vi "ExNCLMult.vi"() -> ()   [LabVIEW 2010]
panel:
  out "Voltage 3":dbl format="%.2f"
  out "Voltage 2":dbl format="%.2f"
  in  "stop":bool
  in  "Number of Detectors (only available for NCL)":u32=1 min=1 max=3 step=1
  in  "Num of Reads to average":u32=1 min=1 step=1
  in  "Gain Range":u32 max=4 step=1
  in  "Integraion / Exposure ms":dbl=1.0 min=1.0 step=1.0 format="%.2f"
  in  "Detector Type":u32=1 min=1 max=3 step=1
  in  "Bi Polar Enable":bool
  in  "High Volts":dbl format="%.2f"
  in  "High Volts Enable":bool
  out "Detector Type":u32
  out "Bi Polar":bool
  out "Gain Value":dbl format="%.2f"
  out "Gain Range":dbl format="%.2f"
  out "Integraion time ms":dbl format="%.2f"
  out "HV Status":bool
  out "HV Volts":dbl format="%.2f"
  out "Get Ave Rds":u32
  out "reserve 2":u32
  out "reserve 1":u32
  out "Voltage 1":dbl format="%.2f"
  out "error out":errorcluster
  in  "error in (no error)":errorcluster
  # "ExNCLMult.vi : shows how to\ncontrol 3 voltages at one time"
  # "1 :  Current\n 2 :  Voltage\n 3 :  Photon Counting"
  # "Minimum is 1.0 ms\nPractical minimum 10.0 ms\nTypical 100.0 ms\nmaximum is 65 sec (65535ms)"
  # "0 : 1x\n1 :  2x\n2 :  4x\n3 : 50x\n4 : 200x"
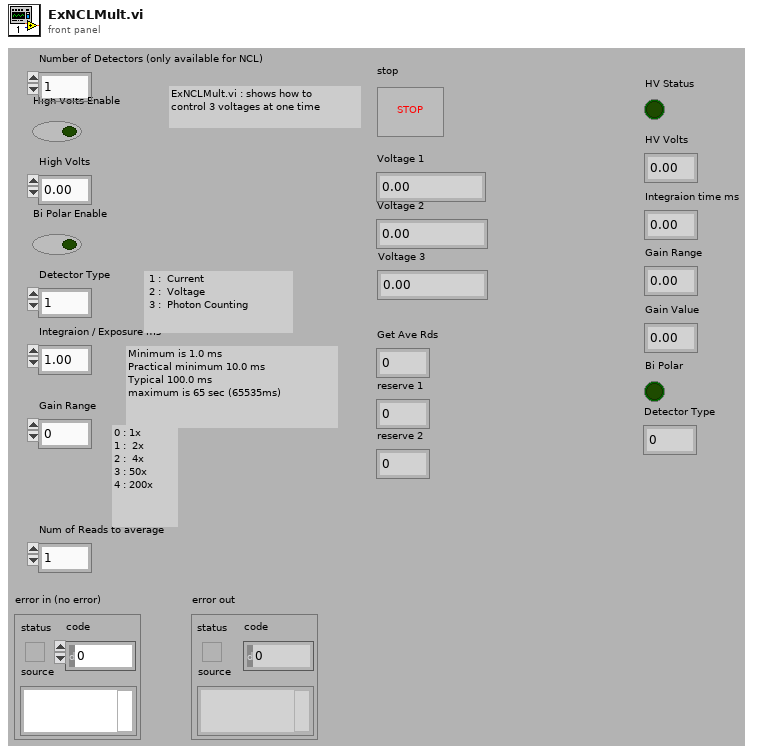
[diagram p1: front panel]
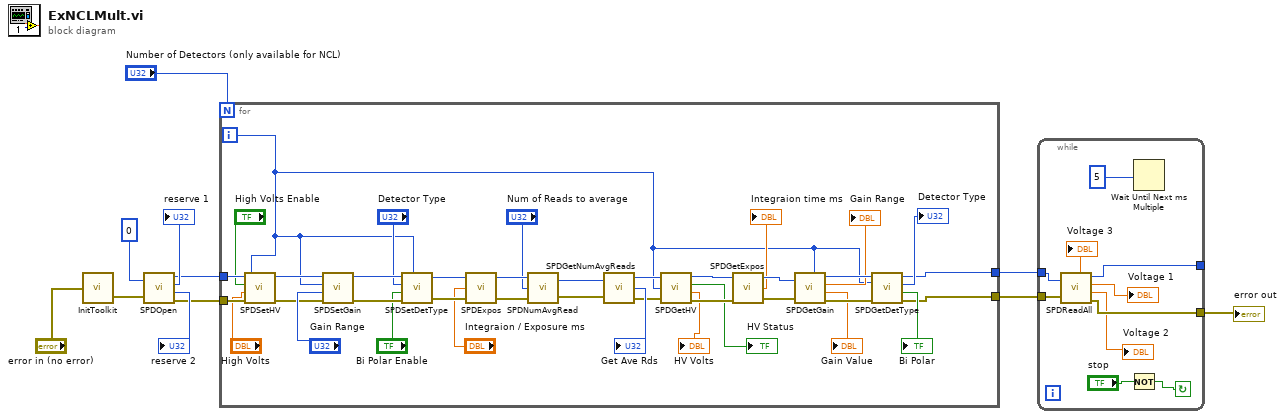
[diagram p0: block diagram]
diagram:
  n1 = call <userlib>:"InitToolkit.vi"("error in"="error in (no error)") -> ("error out"=w10:errorcluster)
  n2 = call <userlib>:"SPDOpen.vi"("Device ID"=0, "error in (no error)"=w10) -> ("SPD Handle"=w5:u32, "reserved 1"=→"reserve 1":u32, "reserved 2"=→"reserve 2":u32, "error out"=w6:errorcluster)
  n3 = for {
    N: "Number of Detectors (only available for NCL)" -> [_]
    tunnel: w6 -> [w33]
    tunnel: w5 -> [w32]
    tunnel: [w14] -> w4
    tunnel: [w13] -> w3
    i -> [w12]
    n4 = call <userlib>:"SPDSetHV.vi"("SPD Handle"=w32, "HV enable/disable"="High Volts Enable", "Volts"="High Volts", "error in (no error)"=w33, "SPD Number"=w12) -> ("SPD Handle"=w27:u32, "error out"=w28:errorcluster)
    n5 = call <userlib>:"SPDSetGain.vi"("error in (no error)"=w28, "Gain Range"="Gain Range", "Detector Number"=w12, "SPD Handle"=w27) -> ("error out"=w26:errorcluster, "SPD Handle"=w25:u32)
    n6 = call <userlib>:"SPDSetDetType.vi"("SPD Handle"=w25, "Detector Type"="Detector Type", "BiPolar switch"="Bi Polar Enable", "error in (no error)"=w26, "SPD Number"=w12) -> ("SPD Handle"=w21:u32, "error out"=w22:errorcluster)
    n7 = call <userlib>:"SPDExpos.vi"("error in (no error)"=w22, "Integration Time (ms)"="Integraion / Exposure ms", "SPD Handle"=w21) -> ("error out"=w19:errorcluster, "SPD Handle"=w18:u32)
    n8 = call <userlib>:"SPDNumAvgRead.vi"("error in (no error)"=w19, "Number to average Reads"="Num of Reads to average", "SPD Handle"=w18) -> ("error out"=w17:errorcluster, "SPD Handle"=w16:u32)
    n9 = call <userlib>:"SPDGetNumAvgReads.vi"("SPD Handle"=w16, "error in (no error)"=w17) -> ("SPD Handle"=w34:u32, "Number of Averages"=→"Get Ave Rds":u32, "error out"=w35:errorcluster)
    n10 = call <userlib>:"SPDGetHV.vi"("SPD Handle"=w34, "Detector Number"=w12, "error in (no error)"=w35) -> ("SPD Handle"=w45:u32, "HV Status (ON/OFF)"=→"HV Status":bool, "HV Volts"=→"HV Volts":dbl, "error out"=w48:errorcluster)
    n11 = call <userlib>:"SPDGetExpos.vi"("error in (no error)"=w48, "SPD Handle"=w45) -> ("error out"=w47:errorcluster, "Integration time in ms"=→"Integraion time ms":dbl, "SPD Handle"=w44:u32)  [unwired: 1 in]
    n12 = call <userlib>:"SPDGetGain.vi"("Detector Number"=w12, "error in (no error)"=w47, "SPD Handle"=w44) -> ("error out"=w46:errorcluster, "Gain value"=→"Gain Value":dbl, "Gain Range"=→"Gain Range":dbl, "SPD Handle"=w43:u32)
    n13 = call <userlib>:"SPDGetDetType.vi"("SPD Handle"=w43, "SPD Number"=w12, "error in (no error)"=w46) -> ("SPD Handle"=w13:u32, "Detector Type"=→"Detector Type":u32, "BiPolar state"=→"Bi Polar":bool, "error out"=w14:errorcluster)
  }
  n14 = while {
    tunnel: w4 -> [w51]
    tunnel: w3 -> [w52]
    tunnel: [w58] -> _
    tunnel: [w57] -> w2
    stop <- w55 continue-if-true
    n15 = call <userlib>:"SPDReadAll.vi"("SPD Handle"=w52, "error in (no error)"=w51) -> ("SPD value 3"=→"Voltage 3":dbl, "SPD Handle"=w58:u32, "SPD value 1"=→"Voltage 1":dbl, "SPD value 2"=→"Voltage 2":dbl, "error out"=w57:errorcluster)  [unwired: 1 out]
    n16 = Not(x="stop") -> (.not. x?=w55:bool)
    n17 = Wait Until Next ms Multiple(millisecond multiple=5) -> ()  [unwired: 1 out]
  }
  "error out" <- w2
